vi "GlobalGetTemperatureCamera.vi"() -> ()   [LabVIEW 2011]
panel:
  out "temperatureCamera":i32(slide) scale=-100.0..20.0
  out "TemperatureStatus":bool
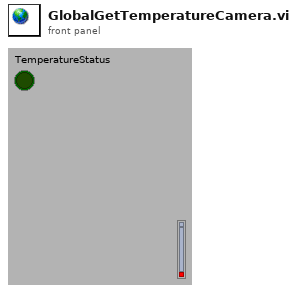
[diagram p1: front panel]
diagram:
